vi "Delete (path).vi"(8 "error in (no error)":errorcluster, 10 "Path":string, 11 "JSON Value in":refnum<class "JSON Value.lvclass">) -> (0 "error out":errorcluster, 3 "JSON Value out":refnum<class "JSON Value.lvclass">)   [LabVIEW 2016, in "JSON Value.lvclass"]
uses:
  JSON Value.lvclass
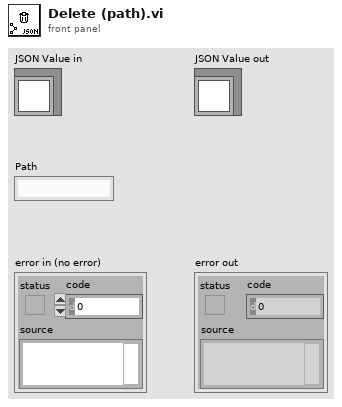
[diagram p1: front panel]
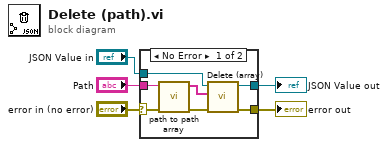
[diagram p0: block diagram]
diagram:
  n1 = case shown="No Error" "error in (no error)" {
    selector: "error in (no error)" -> [w7 w13]
    tunnel: [w11 w14] -> w3
    tunnel: "JSON Value in" -> [w12 w14]
    tunnel: "Path" -> [w9 _]
    tunnel: [w10 w13] -> w1
    frame No Error {
      n2 = call "path to path array.vi"("error in (no error)"=w7, "path"=w9) -> ("error out"=w6:errorcluster, "path array"=w8:string[])  [unwired: 8 in]
      n3 = call "Delete (array).vi"("error in (no error)"=w6, "Path Array"=w8, "JSON Value in"=w12) -> ("error out"=w10:errorcluster, "JSON Value out"=w11:refnum<class "JSON Value.lvclass">)  [unwired: 7 in]
    }
    frame Error {
    }
  }
  "error out" <- w1
  "JSON Value out" <- w3
